vi "Main UI suggestion.vi"() -> ()   [LabVIEW 2017]
uses:
  Spectrometer Utilities/SpectrometerControllerEnum.ctl
  Scripts Actors/MapScriptGFVEnum.ctl
  Microscope/MicroscopeControllerEnum.ctl
  Scripts Actors/MapDryScriptGFVEnum.ctl
panel:
  in  "Add/Remove User 2":bool
  in  "Add/Remove User":bool
  in  "Sample Type":string(combo)="Combo 4" caption="Combo Box"
  in  "Experiment No.":string caption="String"
  in  "Experiment Title":string caption="String"
  out "User Picture":T1(plugin-control)
  in  "User Name":string(combo)="Combo 4" caption="Combo Box"
  in  "Show Spectrometer":bool
  in  "stop":bool
  in  "Script":string(combo)="Combo 1" caption="Combo Box"
  in  "Right Button":bool
  in  "Down Button":bool
  in  "Up Button":bool
  in  "Distance (mm)":i32(slide)=9 min=1 max=10 scale=0.0..10.0
  in  "Left Button":bool
  out "Warnings":string
  out "Suggestions":string
  out "Power\nmeter":bool
  out "Waveplate":bool
  out "Analyzer":bool
  out "Polarizor":bool
  out "Stage":bool
  out "Camera":bool
  out "Status":string
  out "Log":string
  out "System Health Status":string
  # "Yaffe's Lab"
  # "Raman Spectrometer Software - Data Acquisition Software (Weizmann Institute of Science)"
  # "Stage Controller"
  # "Includes icons made by Daniel Bruce (danielbruce.se)"
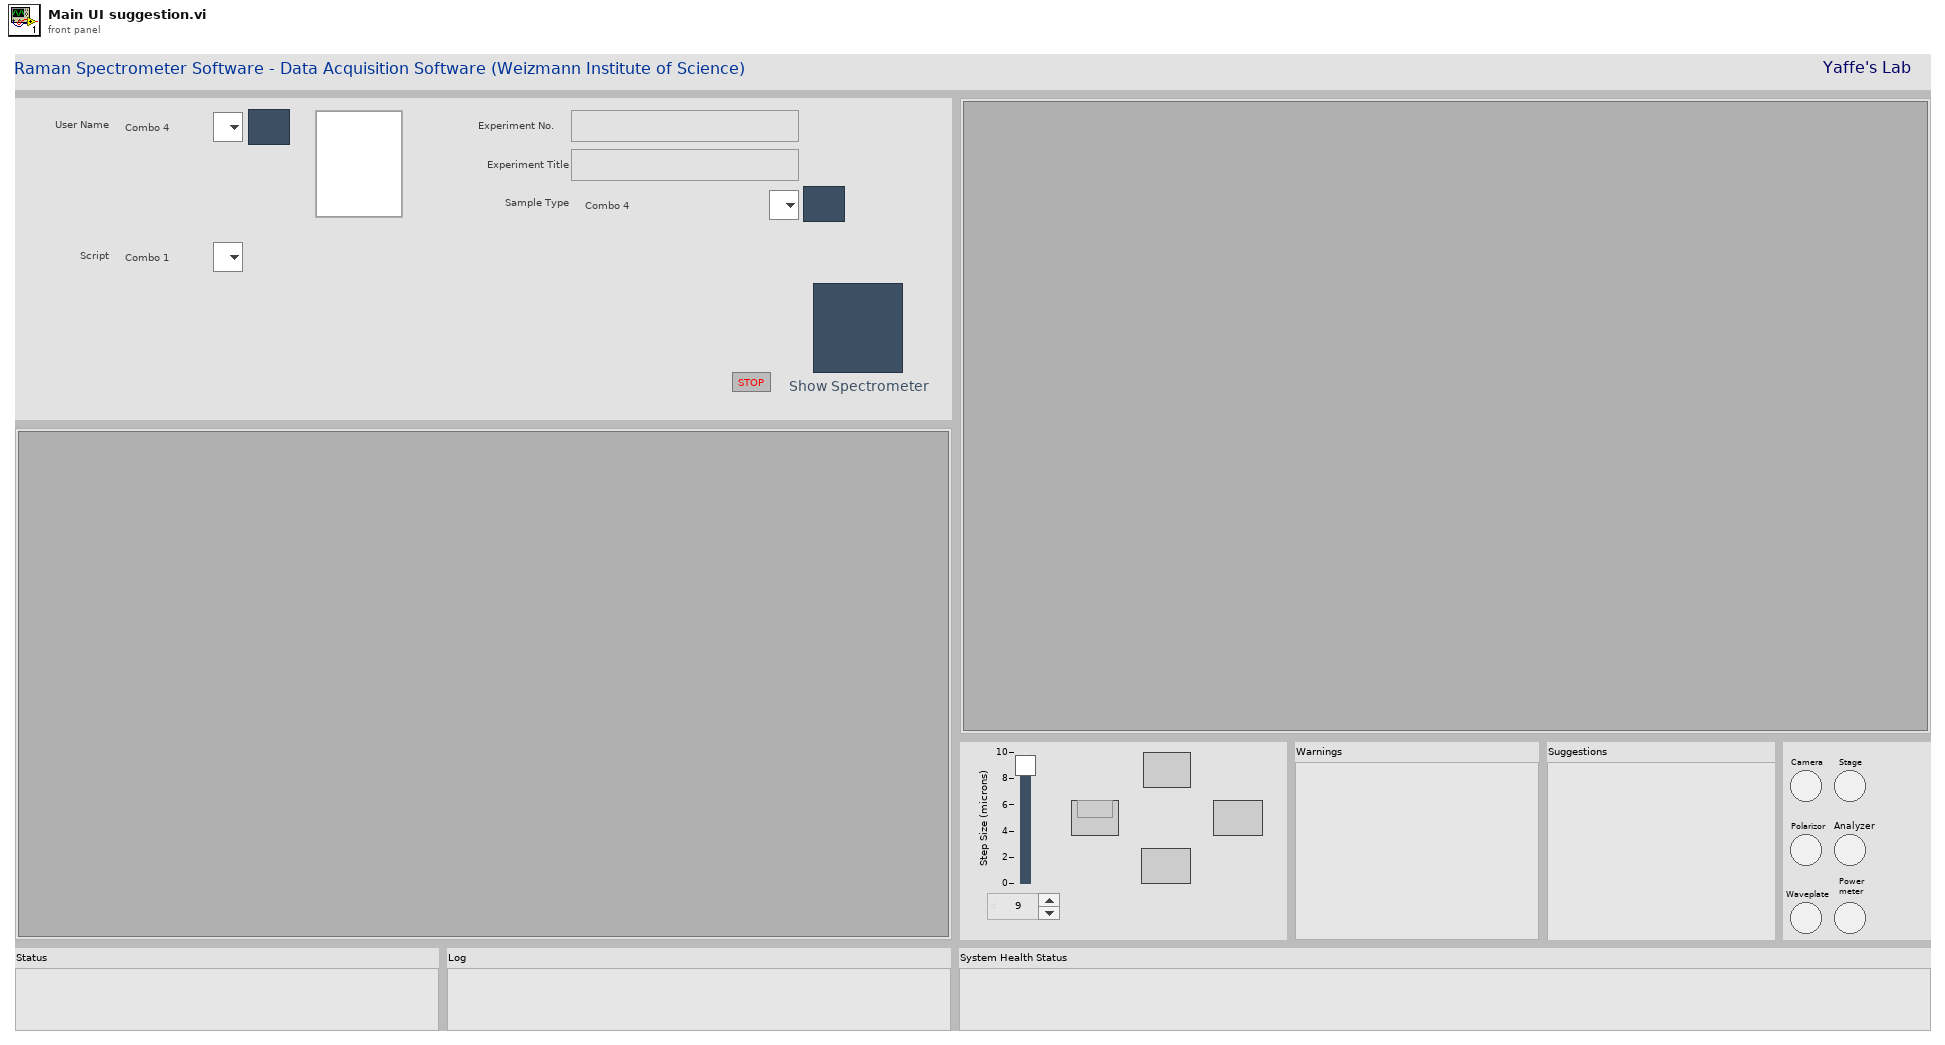
[diagram p1: front panel]
types:
  T1 = typedef "IMAQ Image.ctl" = refnum<image>
  T2 = typedef "MicroscopeControllerEnum.ctl" = enum16{"Init!", "Start!", "Stop!", "GetMicroscopeVIRef", "GetAbsPointsForStage", "InsertCallbackEvent!", "InsertLaserPoint!", "InsertMapPoints!", "InsertMicroscopeImageRef!"}
  T3 = typedef "MapScriptGFVEnum.ctl" = enum16{"Init!", "Stop!", "Start!", "GetMapScriptActorViRef"}
  T4 = typedef "SpectrometerControllerEnum.ctl" = enum16{"Init!", "Start!", "Stop!", "Start New Measurement!", "MeasurementCompleted?", "Update Current Measurement Data", "Get Current Measurement Data!", "GetSpectrometerVIRef!", "Insert Callback Event"}
  T5 = typedef "MapDryScriptGFVEnum.ctl" = enum16{"Init!", "Stop!", "Start!", "GetMapScriptActorViRef"}
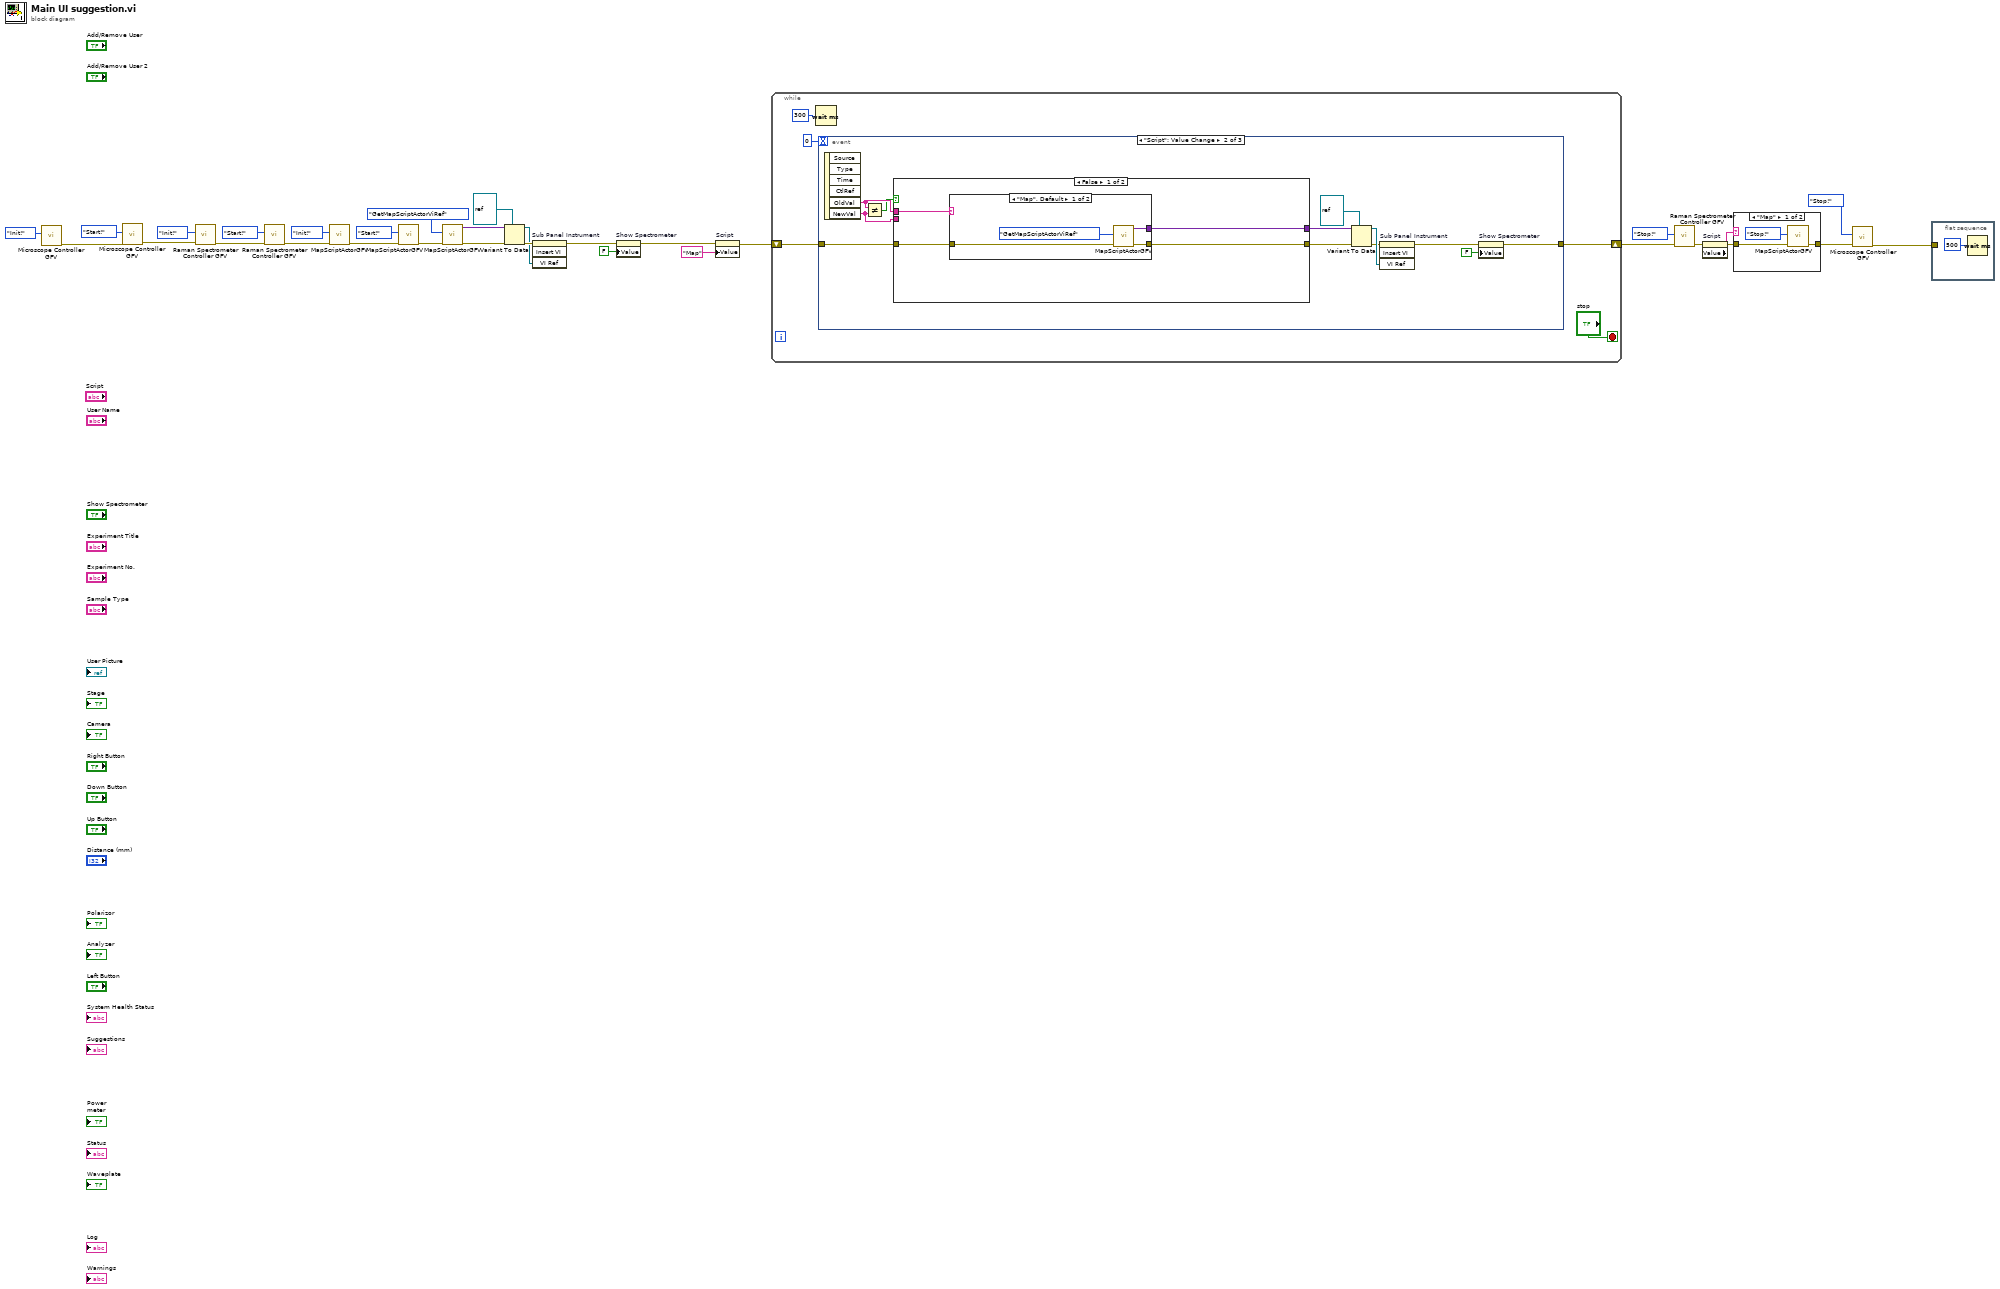
[diagram p0: block diagram]
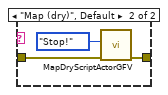
[diagram p2: hidden frame]
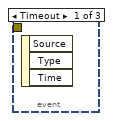
[diagram p3: hidden frame]
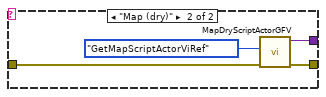
[diagram p4: hidden frame]
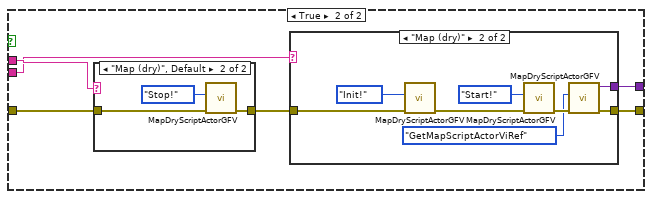
[diagram p5: hidden frame]
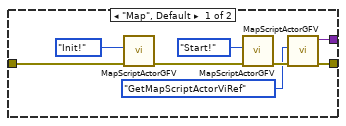
[diagram p6: hidden frame]
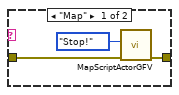
[diagram p7: hidden frame]
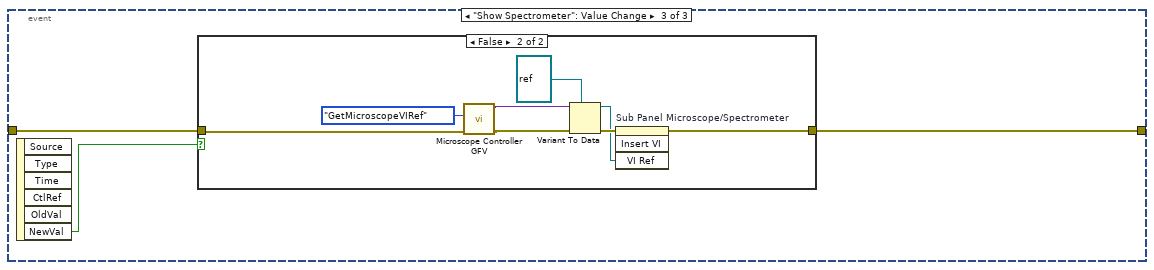
[diagram p8: hidden frame]
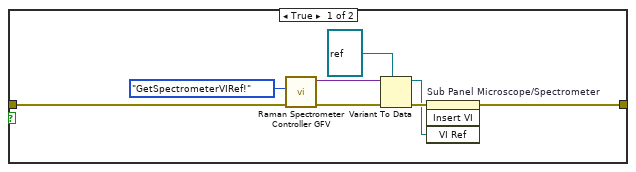
[diagram p9: hidden frame]
diagram:
  n1 = call "Microscope Controller GFV.vi"("MicroscopeEnum"=MicroscopeControllerEnum."Init!") -> ("error out"=w5:errorcluster)  [unwired: 9 in, 1 out]
  n2 = call "Microscope Controller GFV.vi"("error in (no error)"=w5, "MicroscopeEnum"=MicroscopeControllerEnum."Start!") -> ("error out"=w7:errorcluster)  [unwired: 8 in, 1 out]
  n3 = call "Raman Spectrometer Controller GFV.vi"("SpectrometerEnum"=SpectrometerControllerEnum."Init!", "error in (no error)"=w7) -> ("error out"=w31:errorcluster)  [unwired: 7 in, 1 out]
  n4 = call "Raman Spectrometer Controller GFV.vi"("SpectrometerEnum"=SpectrometerControllerEnum."Start!", "error in (no error)"=w31) -> ("error out"=w27:errorcluster)  [unwired: 7 in, 1 out]
  n5 = call "MapScriptActorGFV.vi"("error in (no error)"=w27, "MapScriptEnum"=MapScriptGFVEnum."Init!" ("Enum")) -> ("error out"=w25:errorcluster)  [unwired: 8 in, 1 out]
  n6 = call "MapScriptActorGFV.vi"("error in (no error)"=w25, "MapScriptEnum"=MapScriptGFVEnum."Start!" ("Enum")) -> ("error out"=w12:errorcluster)  [unwired: 8 in, 1 out]
  n7 = call "MapScriptActorGFV.vi"("error in (no error)"=w12, "MapScriptEnum"=MapScriptGFVEnum."GetMapScriptActorViRef") -> ("error out"=w11:errorcluster, "Data Out"=w10:variant)  [unwired: 8 in]
  n8 = Variant To Data(error in=w11, type=refnum<vi> refnum ("vi reference"), Variant=w10) -> (data=w14:refnum<vi>, error out=w15:errorcluster)
  n9 = invoke on="Sub Panel Instrument" class="SubPanel" method="Insert VI"(error in=w15, "VI Ref"=w14) -> (error out=w18:errorcluster)  [unwired: 2 in, 3 out]
  n10 = property on="Show Spectrometer" class="Bool (strict)"(error in=w18, "Value"=FALSE ("Show Spectrometer")) -> (error out=w9:errorcluster)  [unwired: 1 in, 1 out]
  n11 = property on="Script" class="CmbBox"(error in=w9, "Value"="Map" ("Value (Signaling)")) -> (error out=w8:errorcluster)  [unwired: 1 in, 1 out]
  n12 = while {
    shift-right: [w32] -> w23
    shift-left: w8 -> [w34]
    stop <- "stop" stop-if-true
    n13 = Wait (ms)(milliseconds to wait=u32 300) -> ()  [unwired: 1 out]
    n14 = event shown="[1] \"Script\": Value Change" {
      selector: _ -> [_ _ _]
      dyn-events: _ -> [_ _ _]
      timeout: 0 -> [_ _ _]
      tunnel: w34 -> [_ w48 w91]
      tunnel: [_ w37 w90] -> w32
      event Timeout {
        n15 = event-data() -> ()  [unwired: 1 in, 3 out]
      }
      event "Script": Value Change {
        n16 = event-data() -> ("OldVal"=w42:string, "NewVal"=w41:string)  [unwired: 1 in, 4 out]
        n17 = Not Equal?(x=w42, y=w41) -> (x != y?=w40:bool)
        n18 = case shown="False" w40 {
          tunnel: w48 -> [w51 w66]
          tunnel: [w49 w64] -> w44
          tunnel: [w50 w63] -> w43
          tunnel: w42 -> [w52 w62]
          tunnel: w41 -> [_ w61]
          frame False {
            n19 = case shown="\"Map\", Default" w52 {
              tunnel: [w56 w60] -> w50
              tunnel: [w54 w58] -> w49
              tunnel: w51 -> [w53 w57]
              frame "Map", Default {
                n20 = call "MapScriptActorGFV.vi"("error in (no error)"=w53, "MapScriptEnum"=MapScriptGFVEnum."GetMapScriptActorViRef") -> ("error out"=w56:errorcluster, "Data Out"=w54:variant)  [unwired: 8 in]
              }
              frame "Map (dry)" {
                n21 = call "MapDryScriptActorGFV.vi"("error in (no error)"=w57, "MapScriptFGVEnum"=MapDryScriptGFVEnum."GetMapScriptActorViRef") -> ("error out"=w60:errorcluster, "Data Out"=w58:variant)  [unwired: 8 in]
              }
            }
          }
          frame True {
            n22 = case shown="\"Map (dry)\", Default" w62 {
              tunnel: w66 -> [w85 w87]
              tunnel: [w84 w88] -> w65
              frame "Map" {
                n23 = call "MapScriptActorGFV.vi"("error in (no error)"=w85, "MapScriptEnum"=MapScriptGFVEnum."Stop!") -> ("error out"=w84:errorcluster)  [unwired: 8 in, 1 out]
              }
              frame "Map (dry)", Default {
                n24 = call "MapDryScriptActorGFV.vi"("error in (no error)"=w87, "MapScriptFGVEnum"=MapDryScriptGFVEnum."Stop!") -> ("error out"=w88:errorcluster)  [unwired: 8 in, 1 out]
              }
            }
            n25 = case shown="\"Map (dry)\"" w61 {
              tunnel: w65 -> [w74 w82]
              tunnel: [w69 w77] -> w63
              tunnel: [w67 w75] -> w64
              frame "Map", Default {
                n26 = call "MapScriptActorGFV.vi"("error in (no error)"=w74, "MapScriptEnum"=MapScriptGFVEnum."Init!") -> ("error out"=w72:errorcluster)  [unwired: 8 in, 1 out]
                n27 = call "MapScriptActorGFV.vi"("error in (no error)"=w72, "MapScriptEnum"=MapScriptGFVEnum."Start!") -> ("error out"=w70:errorcluster)  [unwired: 8 in, 1 out]
                n28 = call "MapScriptActorGFV.vi"("error in (no error)"=w70, "MapScriptEnum"=MapScriptGFVEnum."GetMapScriptActorViRef") -> ("error out"=w69:errorcluster, "Data Out"=w67:variant)  [unwired: 8 in]
              }
              frame "Map (dry)" {
                n29 = call "MapDryScriptActorGFV.vi"("error in (no error)"=w82, "MapScriptFGVEnum"=MapDryScriptGFVEnum."Init!") -> ("error out"=w80:errorcluster)  [unwired: 8 in, 1 out]
                n30 = call "MapDryScriptActorGFV.vi"("error in (no error)"=w80, "MapScriptFGVEnum"=MapDryScriptGFVEnum."Start!") -> ("error out"=w78:errorcluster)  [unwired: 8 in, 1 out]
                n31 = call "MapDryScriptActorGFV.vi"("error in (no error)"=w78, "MapScriptFGVEnum"=MapDryScriptGFVEnum."GetMapScriptActorViRef") -> ("error out"=w77:errorcluster, "Data Out"=w75:variant)  [unwired: 8 in]
              }
            }
          }
        }
        n32 = Variant To Data(error in=w43, type=refnum<vi> refnum ("vi reference"), Variant=w44) -> (data=w47:refnum<vi>, error out=w46:errorcluster)
        n33 = invoke on="Sub Panel Instrument" class="SubPanel" method="Insert VI"(error in=w46, "VI Ref"=w47) -> (error out=w38:errorcluster)  [unwired: 2 in, 3 out]
        n34 = property on="Show Spectrometer" class="Bool (strict)"(error in=w38, "Value"=FALSE ("Show Spectrometer")) -> (error out=w37:errorcluster)  [unwired: 1 in, 1 out]
      }
      event "Show Spectrometer": Value Change {
        n35 = event-data() -> ("NewVal"=w89:bool)  [unwired: 1 in, 5 out]
        n36 = case shown="False" w89 {
          tunnel: [w92 w104] -> w90
          tunnel: w91 -> [w95 w100]
          frame True {
            n37 = call "Raman Spectrometer Controller GFV.vi"("SpectrometerEnum"=SpectrometerControllerEnum."GetSpectrometerVIRef!", "error in (no error)"=w95) -> ("Data Out"=w98:variant, "error out"=w97:errorcluster)  [unwired: 7 in]
            n38 = Variant To Data(error in=w97, type=refnum<vi> refnum ("vi reference"), Variant=w98) -> (data=w93:refnum<vi>, error out=w94:errorcluster)
            n39 = invoke on="Sub Panel Microscope/Spectrometer" class="SubPanel" method="Insert VI"(error in=w94, "VI Ref"=w93) -> (error out=w92:errorcluster)  [unwired: 2 in, 3 out]
          }
          frame False {
            n40 = call "Microscope Controller GFV.vi"("error in (no error)"=w100, "MicroscopeEnum"=MicroscopeControllerEnum."GetMicroscopeVIRef") -> ("error out"=w102:errorcluster, "Data Out"=w103:variant)  [unwired: 8 in]
            n41 = Variant To Data(error in=w102, type=refnum<vi> refnum ("vi reference"), Variant=w103) -> (data=w105:refnum<vi>, error out=w106:errorcluster)
            n42 = invoke on="Sub Panel Microscope/Spectrometer" class="SubPanel" method="Insert VI"(error in=w106, "VI Ref"=w105) -> (error out=w104:errorcluster)  [unwired: 2 in, 3 out]
          }
        }
      }
    }
  }
  n43 = call "Raman Spectrometer Controller GFV.vi"("SpectrometerEnum"=SpectrometerControllerEnum."Stop!", "error in (no error)"=w23) -> ("error out"=w20:errorcluster)  [unwired: 7 in, 1 out]
  n44 = property on="Script" class="CmbBox"(error in=w20) -> (error out=w19:errorcluster, "Value"=w22:string)  [unwired: 1 in, 1 out]
  n45 = case shown="\"Map\"" w22 {
    tunnel: w19 -> [w110 w112]
    tunnel: [w109 w113] -> w3
    frame "Map" {
      n46 = call "MapScriptActorGFV.vi"("error in (no error)"=w110, "MapScriptEnum"=MapScriptGFVEnum."Stop!") -> ("error out"=w109:errorcluster)  [unwired: 8 in, 1 out]
    }
    frame "Map (dry)", Default {
      n47 = call "MapDryScriptActorGFV.vi"("error in (no error)"=w112, "MapScriptFGVEnum"=MapDryScriptGFVEnum."Stop!") -> ("error out"=w113:errorcluster)  [unwired: 8 in, 1 out]
    }
  }
  n48 = call "Microscope Controller GFV.vi"("error in (no error)"=w3, "MicroscopeEnum"=MicroscopeControllerEnum."Stop!") -> ("error out"=w2:errorcluster)  [unwired: 8 in, 1 out]
  n49 = flat-sequence {
    tunnel: w2 -> [_]
    frame #0 {
      n50 = Wait (ms)(milliseconds to wait=u32 500) -> ()  [unwired: 1 out]
    }
  }
